vi "Send Ping Actor.vi"(7 "Priority":T1 caption="Message Priority (Normal)", 8 "error in (no error)":errorcluster, 10 "Actor":refnum<class "Message Enqueuer.lvclass">, 11 "Message Enqueuer in":refnum<class "Message Enqueuer.lvclass">) -> (0 "error out":errorcluster, 3 "Message Enqueuer out":refnum<class "Message Enqueuer.lvclass">)   [LabVIEW 2020, in "Monitored Actor.lvlib" / "Ping Actor Msg.lvclass"]
doc: "Sends the <b>Monitored Actor.lvlib:Ping Actor Msg.lvclass</b> message.\n\nThis message will call <b>Ping Actor.vi</b> on the <b>Monitored Actor.lvlib:Actor Monitor.lvclass</b> actor.\n\n<b>Ping Actor.vi Description</b>\nSends a ping message to the actor\n\nCopyright: MGI 2016\nAuthor: Derek Trepanier"
uses:
  <vilib>/MGI/Monitored Actor/Actor Monitor/Actor Monitor Messages/Ping Actor Msg/Ping Actor Msg.lvclass
  <vilib>/ActorFramework/Message Enqueuer/Message Enqueuer.lvclass
  <vilib>/ActorFramework/Message Enqueuer/Message Priority.ctl
  C:/Program Files/National Instruments/LabVIEW 2020/vi.lib/ActorFramework/Message/Message.lvclass
  <vilib>/MGI/Monitored Actor/Actor Monitor/Actor Monitor Messages/Ping Actor Msg/Ping Actor Msg.lvclass/Ping Actor Msg.ctl
  <vilib>/ActorFramework/Message Enqueuer/Message Enqueuer.lvclass/Message Enqueuer.ctl
  <vilib>/ActorFramework/Message Priority Queue/Priority Enqueue.vi
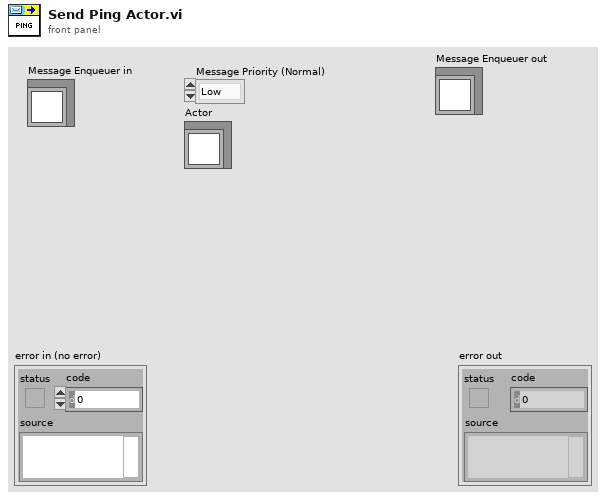
[diagram p1: front panel]
types:
  T1 = typedef "Actor Framework.lvlib/Message Enqueuer.lvclass/Message Priority.ctl" = enum16{"Low", "Normal", "High"}
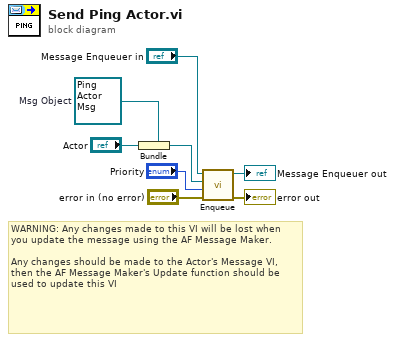
[diagram p0: block diagram]
diagram:
  w7 = refnum<class "Ping Actor Msg.lvclass"> refnum  # Msg Object
  # "WARNING: Any changes made to this VI will be lost when you update the message using the AF Message Maker.\n\nAny changes should be made to the Actor's Message VI, then the AF Message Maker's Update function should be used to update this VI"
  n1 = Bundle(cluster=w7, "Actor") -> (w2:refnum<class "Ping Actor Msg.lvclass">)
  n2 = call <vilib>:"Enqueue.vi"("error in (no error)"="error in (no error)", "Message Priority (Normal)"="Priority", "Message"=w2, "Message Enqueuer in"="Message Enqueuer in") -> ("error out"=→"error out":errorcluster, "Message Enqueuer out"=→"Message Enqueuer out":refnum<class "Message Enqueuer.lvclass">)  [unwired: 6 in]
